vi "Find COM Ports.vi"(11 "Search Mode":T1 items=["Canonical Names Only"=0, "Aliases Only"=2, "Include Matching Aliases"=3, "Include All Aliases"=4]) -> (2 "COM List":string[](array[string]), 3 "find list":string[](array[string]))   [LabVIEW 2017]
uses:
  <vilib>/Instr/_visa.llb/VISA Find Search Mode.ctl
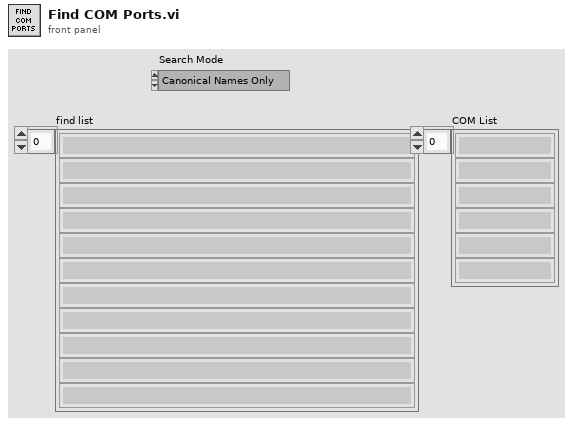
[diagram p1: front panel]
types:
  T1 = typedef "VISA Find Search Mode.ctl" = u32
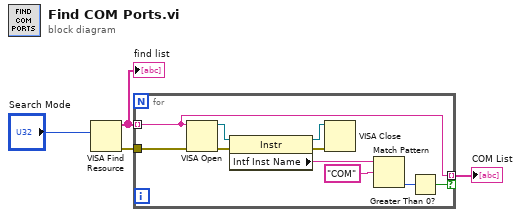
[diagram p0: block diagram]
diagram:
  n1 = VISA Find Resource(10:"Search Mode") -> (0:w4:errorcluster, 3:w3:string[])  [unwired: 2 in, 1 out]
  "find list" <- w3
  n2 = for {
    tunnel: w4 -> [w7]
    tunnel: w3 -> [w6] mode=indexing
    tunnel: [w6] -> w2 mode=indexing if=w5
    n3 = VISA Open(error in (no error)=w7, VISA resource name=w6) -> (VISA resource name=w14:refnum<visa-resource-name>, error out=w13:errorcluster)  [unwired: 3 in]
    n4 = property class="Instr"(reference=w14, error in=w13) -> (reference out=w11:refnum<visa-resource-name>, error out=w12:errorcluster, "Intf Inst Name"=w9:string)
    n5 = VISA Close(VISA resource name=w11, error in (no error)=w12) -> ()  [unwired: 1 out]
    n6 = Match Pattern(string=w9, regular expression="COM") -> (offset past match=w8:i32)  [unwired: 1 in, 3 out]
    n7 = Greater Than 0?(x=w8) -> (x > 0?=w5:bool)
  }
  "COM List" <- w2
